vi "pp_trialTypes_makeWeightedCodeList.vi"(10 "Trial Replication Factor":i32=1 min=1, 11 "Trial Types":T1(array[cluster])=[{"Trial Code"=1, "Trial Type"=enum."GO", "Trial Weight"=1, "Stim Type"=enum."Pure Tone", "Stim Dur (s)"=0.0, "Stim P1"=0.0, "Stim P2"=0.0}, {"Trial Code"=2, "Trial Type"=enum."NOGO", "Trial Weight"=2, "Stim Type"=enum."Pure Tone", "Stim Dur (s)"=0.0, "Stim P1"=0.0, "Stim P2"=0.0}, {"Trial Code"=3, "Trial Type"=enum."TEST", "Trial Weight"=3, "Stim Type"=enum."Pure Tone", "Stim Dur (s)"=0.0, "Stim P1"=0.0, "Stim P2"=0.0}] {"Stim P2" min=0.0; "Trial Weight" step=1; "Stim P1" min=0.0; "Stim Dur (s)" min=0.0; "Trial Code" min=1 step=1}) -> (3 "Weighted Code List":i32[](array[numeric]), 5 "Weighted Code List Length":i32)   [LabVIEW 2013]
uses:
  labolabo/array/impl/NullArray_I.vi
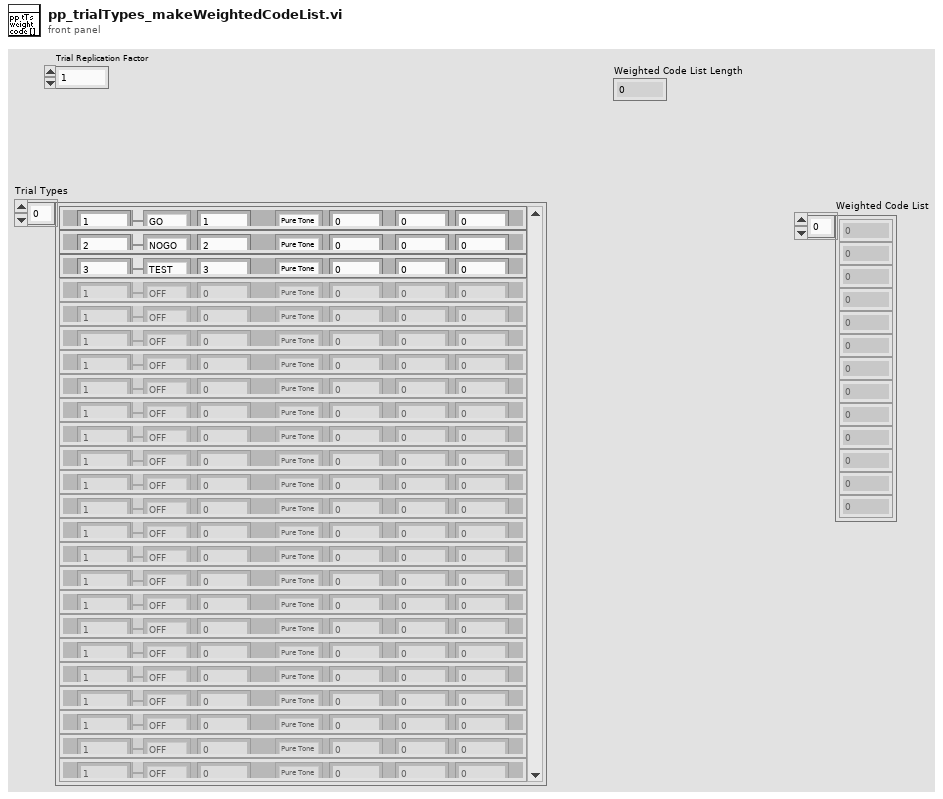
[diagram p1: front panel]
types:
  T1 = cluster{"Trial Code":u16, "Trial Type":enum16{"OFF", "GO", "NOGO", "TEST"}, "Trial Weight":u32, "Stim Type":enum16{"Pure Tone", "FM Sweep"}, "Stim Dur (s)":dbl, "Stim P1":dbl, "Stim P2":dbl}[]
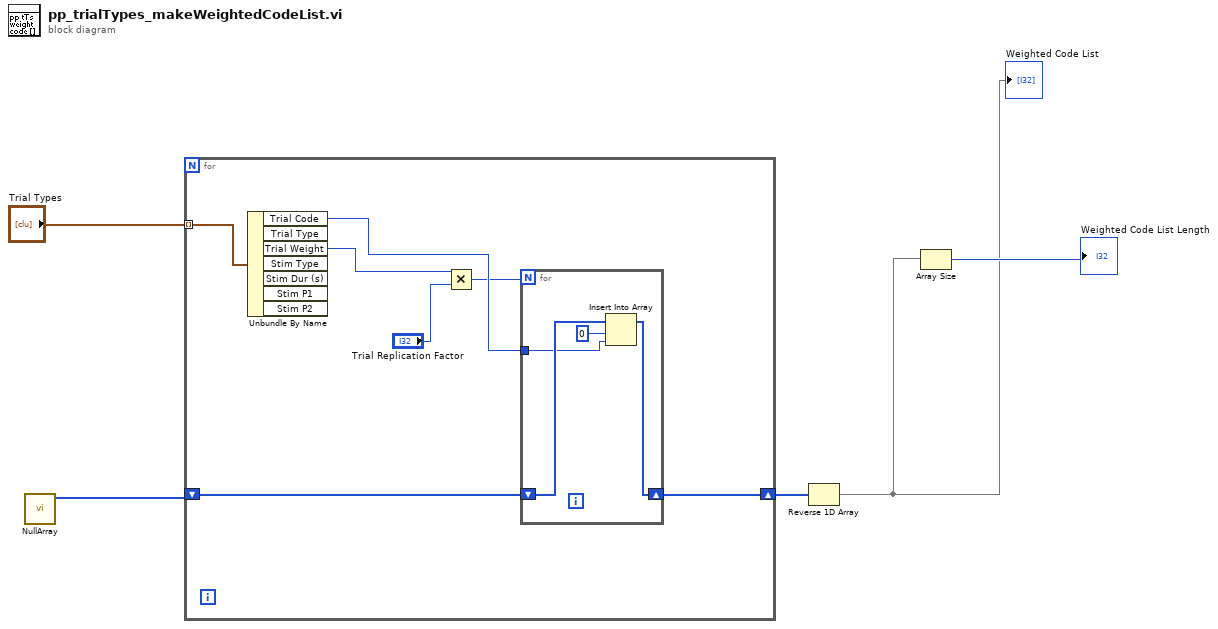
[diagram p0: block diagram]
diagram:
  n1 = call-poly "NullArray.vi"() -> ("Null Array"=w3:i32[])  [unwired: 11 in]
  n2 = for {
    tunnel: "Trial Types" -> [w10] mode=indexing
    shift-right: [w11] -> w4
    shift-left: w3 -> [w12]
    n3 = Unbundle By Name(w10) -> ("Trial Code"=w8:u16, "Trial Weight"=w9:u32)  [unwired: 5 out]
    n4 = Multiply(x=w9, y="Trial Replication Factor") -> (x*y=w6:u32)
    n5 = for {
      N: w6 -> [_]
      shift-right: [w13] -> w11
      shift-left: w12 -> [w15]
      tunnel: w8 -> [w14]
      n6 = Insert Into Array(array=w15, index=0, new element=w14) -> (w13:i32[])
    }
  }
  n7 = Reverse 1D Array(array=w4) -> (reversed array=w1:i32[])
  "Weighted Code List" <- w1
  n8 = Array Size(array=w1) -> (size(s)=→"Weighted Code List Length":i32)
